vi "SizePrompt.vi"(9 "Container State":T1, 11 "Display State In in":T2) -> (3 "Display State In out":T2)   [LabVIEW 2019, in "ExpandVertical.xctl"]
uses:
  ExpandVertical.xctl
  State.ctl
  <vilib>/_xctls/Container State.ctl
  <vilib>/_xctls/XControlSupport.lvlib
panel:
  in  "Cancel":bool
  in  "OK":bool
  in  "Pixels":i16
  # "How much should the FP expand?"
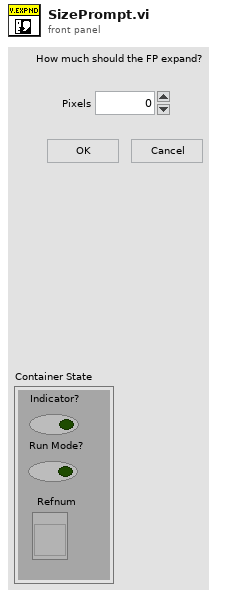
[diagram p1: front panel]
types:
  T1 = typedef "XControlSupport.lvlib/Container State.ctl" = cluster{"Indicator?":bool, "Run Mode?":bool, " Refnum":refnum<vi>}
  T2 = typedef "ExpandVertical.xctl/State.ctl" = cluster{"Size":i16, "Expanded":bool}
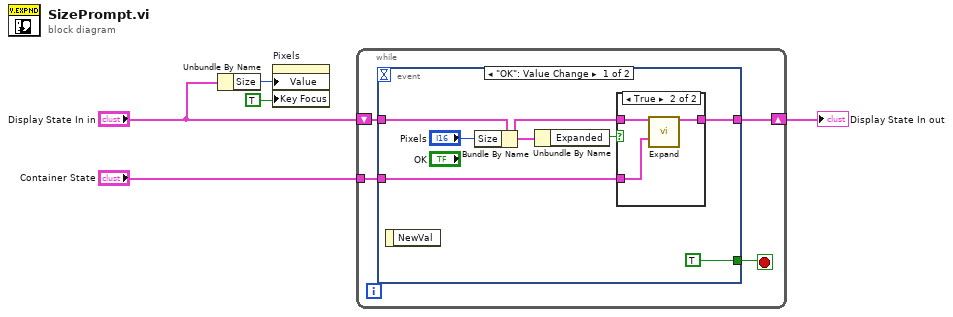
[diagram p0: block diagram]
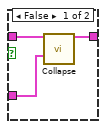
[diagram p2: hidden frame]
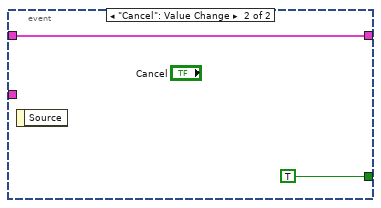
[diagram p3: hidden frame]
diagram:
  n1 = Unbundle By Name("Display State In in") -> ("Size"=w3:i16)
  n2 = property on="Pixels" class="DigNum (strict)"("Value"=w3, "Key Focus"=TRUE) -> ()  [unwired: 2 in, 2 out]
  n3 = while {
    shift-right: [w8] -> w5
    shift-left: "Display State In in" -> [w9]
    tunnel: "Container State" -> [w6]
    stop <- w7 stop-if-true
    n4 = event shown="[0] \"OK\": Value Change" {
      selector: _ -> [_ _]
      dyn-events: _ -> [_ _]
      timeout: _ -> [_ _]
      tunnel: w9 -> [w15 w24]
      tunnel: [w10 w24] -> w8
      tunnel: [TRUE TRUE] -> w7
      tunnel: w6 -> [w13 _]
      event "OK": Value Change {
        n5 = event-data() -> ()  [unwired: 1 in, 1 out]
        n6 = Bundle By Name(cluster=w15, "Size"="Pixels") -> (w12:T2)
        n7 = Unbundle By Name(w12) -> ("Expanded"=w11:bool)
        n8 = case shown="True" w11 {
          tunnel: w13 -> [w17 w22]
          tunnel: w12 -> [w19 w21]
          tunnel: [w18 w20] -> w10
          frame False {
            n9 = call "Collapse.vi"("Display State In"=w19, "Container State"=w17) -> ("Display State Out"=w18:T2)  [unwired: 12 in, 1 out]
          }
          frame True {
            n10 = call "Expand.vi"("Display State In"=w21, "Container State"=w22) -> ("Display State Out"=w20:T2)  [unwired: 12 in, 1 out]
          }
        }
      }
      event "Cancel": Value Change {
        n11 = event-data() -> ()  [unwired: 1 in, 1 out]
      }
    }
  }
  "Display State In out" <- w5
